vi "Pulse Train Generator.vi"() -> ()   [LabVIEW 2009]
uses:
  <vilib>/DAQmx/create/channels.llb/DAQmx Create Channel (CO-Pulse Generation-Frequency).vi
panel:
  in  "initial delay":dbl=0.25 format="%.6f"
  in  "idle state":i32(ring)=10214 items=["High"=10192, "Low"=10214]
  in  "counter":tag="Dev1/ctr0"
  in  "frequency":dbl=1.0 format="%.6f"
  in  "duty cycle":dbl=0.5 format="%.6f"
  in  "stop":bool
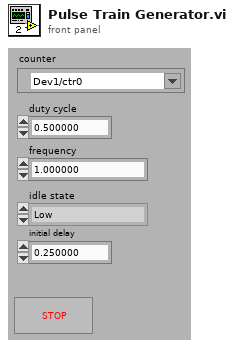
[diagram p1: front panel]
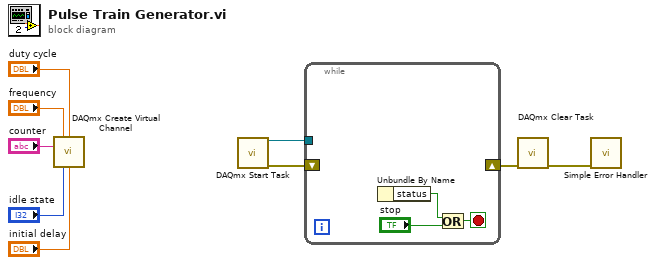
[diagram p0: block diagram]
diagram:
  n1 = call-poly <vilib>:"DAQmx Create Virtual Channel.vi"("frequency"="frequency", "duty cycle"="duty cycle", "counter"="counter", "idle state"="idle state", "initial delay"="initial delay") -> ()  [unwired: 9 in, 2 out]
  n2 = call <vilib>:"DAQmx Start Task.vi"() -> ("task out"=w9:refnum<k21>, "error out"=w8:errorcluster)  [unwired: 14 in]
  n3 = while {
    tunnel: w9 -> [_]
    shift-right: [_] -> w7
    shift-left: w8 -> [_]
    stop <- w10 stop-if-true
    n4 = Unbundle By Name "Unbundle By Name"() -> ("status"=w12:bool)  [unwired: 1 in]
    n5 = Or(x=w12, y="stop") -> (x .or. y?=w10:bool)
  }
  n6 = call <vilib>:"DAQmx Clear Task.vi"("error in"=w7) -> ("error out"=w6:errorcluster)  [unwired: 14 in]
  n7 = call <vilib>:"Simple Error Handler.vi"("error in (no error)"=w6) -> ()  [unwired: 4 in, 5 out]
